vi "format SQLite3 error.vi"(6 "SQLite3LV Connection result":i32, 7 "ppDb":i64 format="%.0x", 8 "error in (no error)":errorcluster, 10 "psqlite":refnum<class "sqlite3.lvclass">, 11 "extra message":string) -> (0 "error out":errorcluster)   [LabVIEW 2014, in "SQLite3LV.lvlib"]
uses:
  SQLite3LV.lvlib
  SQLite3 Class/sqlite3.lvclass
  SQLite3 Class/sqlite3.lvclass/sqlite3.ctl
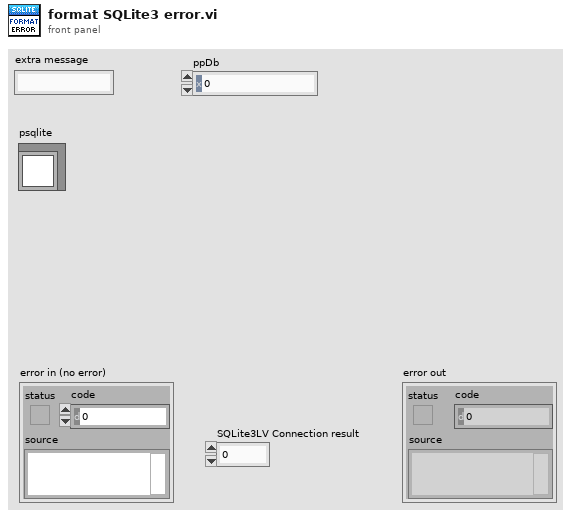
[diagram p1: front panel]
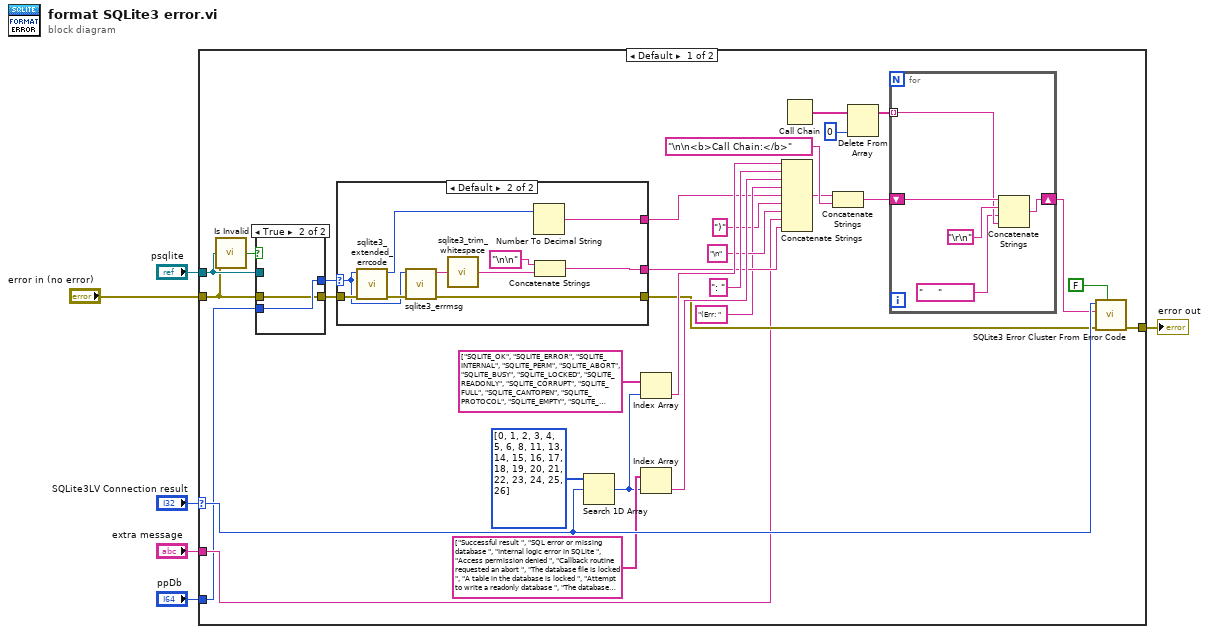
[diagram p0: block diagram]
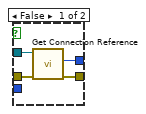
[diagram p2: hidden frame]
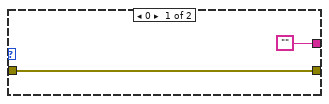
[diagram p3: hidden frame]
diagram:
  n1 = case shown="Default" "SQLite3LV Connection result" {
    selector: "SQLite3LV Connection result" -> [w35 _]
    tunnel: [w28 w60] -> w5
    tunnel: "error in (no error)" -> [w9 w60]
    tunnel: "psqlite" -> [w10 _]
    tunnel: "extra message" -> [w17 _]
    tunnel: "ppDb" -> [w7 _]
    frame Default {
      n2 = call "Is Invalid.vi"("error in (no error)"=w9, "SQLite3LV Connection in"=w10) -> ("not a database"=w8:bool)  [unwired: 2 in, 1 out]
      n3 = case shown="True" w8 {
        tunnel: [w40 w42] -> w12
        tunnel: [w39 w41] -> w11
        tunnel: w10 -> [w38 _]
        tunnel: w9 -> [w37 w41]
        tunnel: w7 -> [_ w42]
        frame False {
          n4 = call "Get Connection Reference.vi"("error in (no error)"=w37, "SQLite3LV Connection in"=w38) -> ("error out"=w39:errorcluster, "ppDb"=w40:i64)  [unwired: 7 in, 1 out]
        }
        frame True {
        }
      }
      n5 = case shown="Default" w12 {
        selector: w12 -> [_ w47]
        tunnel: ["" w51] -> w18
        tunnel: w11 -> [w43 w49]
        tunnel: [w43 w54] -> w19
        tunnel: [_ w45] -> w13
        frame 0 {
        }
        frame Default {
          n6 = call "sqlite3_extended_errcode.vi"("error in (no error)"=w49, "psqlite"=w47) -> ("error out"=w48:errorcluster, "extended error code"=w46:i32)  [unwired: 8 in]
          n7 = call "sqlite3_errmsg.vi"("error in (no error)"=w48, "psqlite"=w47) -> ("error out"=w54:errorcluster, "return type"=w53:string)  [unwired: 8 in]
          n8 = call "sqlite3_trim_whitespace.vi"("string"=w53) -> ("trimmed string"=w50:string)  [unwired: 1 in]
          n9 = Number To Decimal String(number=w46) -> (decimal integer string=w45:string)  [unwired: 1 in]
          n10 = Concatenate Strings("\n\n" ("string"), w50) -> (w51:string)
        }
      }
      n11 = Search 1D Array(1D array=i32[] [0, 1, 2, 3, 4, 5, 6, 8, 11, 13, 14, 15, 16, 17, 18, 19, 20, 21, 22, 23, 24, 25, 26] ("values"), element=w35) -> (index of element=w32:i32)  [unwired: 1 in]
      n12 = Index Array(array=string[] ["SQLITE_OK", "SQLITE_ERROR", "SQLITE_INTERNAL", "SQLITE_PERM", "SQLITE_ABORT", "SQLITE_BUSY", "SQLITE_LOCKED", "SQLITE_READONLY", "SQLITE_CORRUPT", "SQLITE_FULL", "SQLITE_CANTOPEN", "SQLITE_PROTOCOL", "SQLITE_EMPTY", "SQLITE_SCHEMA", "SQLITE_TOOBIG", "SQLITE_CONSTRAINT", "SQLITE_MISMATCH", "SQLITE_MISUSE", "SQLITE_NOLFS", "SQLITE_AUTH", "SQLITE_FORMAT", "SQLITE_RANGE", "SQLITE_NOTADB"] ("strings"), index=w32) -> (element=w31:string)
      n13 = Index Array(array=string[] ["Successful result ", "SQL error or missing database ", "Internal logic error in SQLite ", "Access permission denied ", "Callback routine requested an abort ", "The database file is locked ", "A table in the database is locked ", "Attempt to write a readonly database ", "The database disk image is malformed ", "Insertion failed because database is full ", "Unable to open the database file ", "Database lock protocol error ", "Database is empty ", "The database schema changed ", "String or BLOB exceeds size limit ", "Abort due to constraint violation ", "Data type mismatch ", "Library used incorrectly ", "Uses OS features not supported on host ", "Authorization denied ", "Auxiliary database format error ", "2nd parameter to sqlite3_bind out of range ", "File opened that is not a database file "] ("descriptions"), index=w32) -> (element=w30:string)
      n14 = Concatenate Strings(w31, ": " ("string"), w30, "(Err: " ("string"), w13, ")" ("string"), "\n" ("string"), w17, w18) -> (w21:string)
      n15 = Call Chain() -> (call chain=w22:string[])
      n16 = Concatenate Strings(w21, "\n\n<b>Call Chain:</b>" ("call chain header")) -> (w23:string)
      n17 = Delete From Array(array=w22, index=0) -> (array with subset deleted=w25:string[])  [unwired: 1 in, 1 out]
      n18 = for {
        tunnel: w25 -> [w56] mode=indexing
        shift-right: [w59] -> w20
        shift-left: w23 -> [w57]
        n19 = Concatenate Strings(w57, "\r\n", "     ", w56) -> (w59:string)
      }
      n20 = call "SQLite3 Error Cluster From Error Code.vi"("show call chain? (False)"=FALSE, "error in (no error)"=w19, "error message (\"\")"=w20, "error code (0)"=w35) -> ("error out"=w28:errorcluster)  [unwired: 5 in]
    }
    frame 0, 100, 101 {
    }
  }
  "error out" <- w5
